vi "_setVIRef.vi"(7 "parentURL":string, 8 "error in (no error)":errorcluster, 10 "Refnum":refnum<vi>, 11 "TagDB in":T1) -> (0 "error out":errorcluster, 2 "URL":string, 3 "TagDB out":T1)   [LabVIEW 2014, in "RefManager(dev).lvlib"]
uses:
  RefManager(dev).lvlib
  <userlib>/_NEVSTOP/TagDB/Core/tagDB_Def.ctl
  <userlib>/_NEVSTOP/TagDB/Core/_Support/Access/_setAnything.vi
  <userlib>/_NEVSTOP/TagDB/Core/_XNode/tagDB_setValue.xnode/tagDB_setValue.xnode
  <userlib>/_NEVSTOP/TagDB/Core/TagDB.lvlib
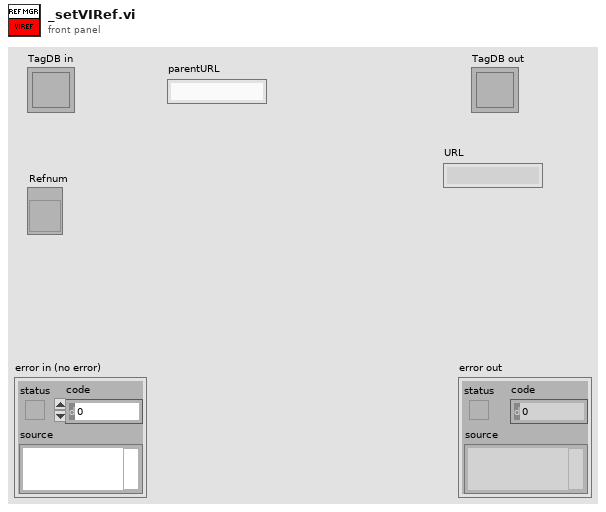
[diagram p1: front panel]
types:
  T1 = typedef "TagDB.lvlib/tagDB_Def.ctl" = refnum<k1>
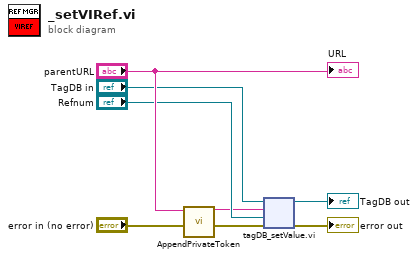
[diagram p0: block diagram]
diagram:
  n1 = call <userlib>:"AppendPrivateToken.vi"("DataURL"="parentURL") -> ("String"=w3:string)  [unwired: 10 in]
  n2 = xnode "tagDB_setValue.vi"("DB Ref"="TagDB in", "name"=w3, "value"="Refnum", "Error In"="error in (no error)") -> ("DB Ref(dup)"=→"TagDB out":T1, "Error Out"=→"error out":errorcluster)  [unwired: 1 out]
  "URL" <- "parentURL"
